vi "Insert Data to DVR.vi"(8 "Data Available":bool, 9 "Sample Count":u32, 10 "New Data":u32[](array[numeric]), 11 "Probe Data Array DVR":refnum<data-value>) -> (1 "Sample Count out":u32)   [LabVIEW 2015, in "Tool Interface.lvlib"]
uses:
  Tool Interface.lvlib
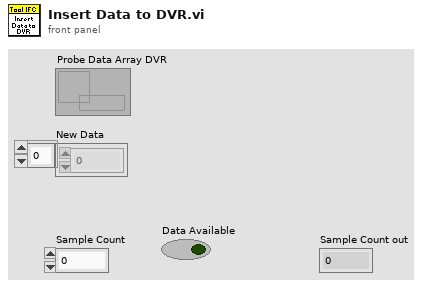
[diagram p1: front panel]
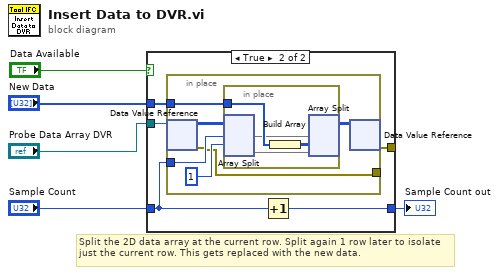
[diagram p0: block diagram]
diagram:
  # "Split the 2D data array at the current row. Split again 1 row later to isolate just the current row. This gets replaced with the new data."
  n1 = case shown="True" "Data Available" {
    tunnel: "New Data" -> [_ w11]
    tunnel: "Probe Data Array DVR" -> [_ w10]
    tunnel: "Sample Count" -> [w6 w9]
    tunnel: [w6 w8] -> w4
    tunnel: [_ w7] -> _
    frame False {
    }
    frame True {
      n2 = in-place {
        in-place-border: w11 -> [w17]
        in-place-border: w9 -> [w14]
        in-place-border: [w12] -> _
        n3 = in-place-dvr #1(w10) -> (w16:u32[][], w12:errorcluster)
        n4 = in-place {
          in-place-border: w17 -> [w21]
          n5 = in-place-split #2(w16, w14, 1) -> (w20:u32[][], w19:u32[][])  [unwired: 1 out]
          n6 = Build Array(w21) -> (w18:u32[][])
          n7 = in-place-split #2(w20, w18, w19) -> (w15:u32[][])  [unwired: 2 out]
        }
        n8 = in-place-dvr #1(w15) -> (w7:errorcluster)  [unwired: 1 out]
      }
      n9 = Increment(x=w9) -> (x+1=w8:u32)
    }
  }
  "Sample Count out" <- w4
